vi "test pass channel to async vis.vi"(11 "Test Case In":refnum<class "Tests Event MessengerM.lvclass">) -> (0 "error out":errorcluster, 3 "Test Case Out":refnum<class "Tests Event MessengerM.lvclass">)   [LabVIEW 2020, in "Tests Event MessengerM.lvclass"]
uses:
  Tests Event MessengerM.lvclass
  C:/Program Files/National Instruments/LabVIEW 2025/vi.lib/Astemes/LUnit/Test Case.lvclass
  <vilib>/Astemes/LUnit/Test Case.lvclass/Test Case.ctl
  Tests Event MessengerM.lvclass/Tests Event MessengerM.ctl
  source/Event MessengerM.lvlib
  <vilib>/Astemes/LUnit/Test Case.lvclass
  C:/Program Files/National Instruments/LabVIEW 2025/vi.lib/Astemes/LUnit/LUnit Runnable.lvclass
  D:/git/Event-MessengerM-Channel-Wire/tests/Tests Event MessengerM/Tests Event MessengerM.lvclass
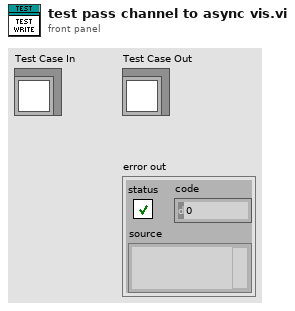
[diagram p1: front panel]
types:
  T1 = typedef "Event MessengerM.lvlib/))Channel.ctl" = refnum<queue>
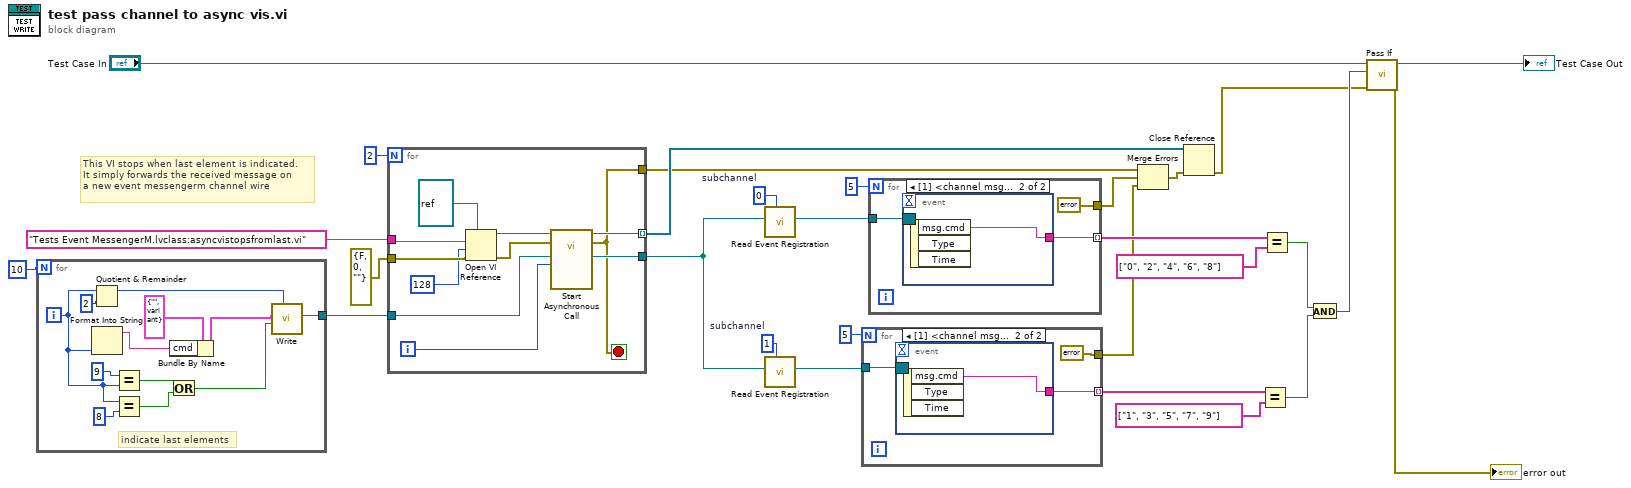
[diagram p0: block diagram]
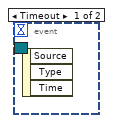
[diagram p2: hidden frame]
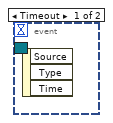
[diagram p3: hidden frame]
diagram:
  w3 = 1  # subchannel
  w4 = 0  # subchannel
  # "This VI stops when last element is indicated.\nIt simply forwards the received message on\na new event messengerm channel wire"
  n1 = for {
    N: 10 -> [_]
    tunnel: [w40] -> w12
    i -> [w30]
    # "indicate last elements"
    n2 = Quotient & Remainder(x=w30, y=2) -> (x-y*floor(x/y)=w38:i32)  [unwired: 1 out]
    n3 = Format Into String(w30) -> (resulting string=w35:string)  [unwired: 3 in, 1 out]
    n4 = Equal?(x=9, y=w30) -> (x = y?=w33:bool)
    n5 = Equal?(x=w30, y=8 ("x")) -> (x = y?=w29:bool)
    n6 = Or(x=w33, y=w29) -> (x .or. y?=w32:bool)
    n7 = Bundle By Name(cluster=cluster{"cmd":string, "data":variant} {"cmd"="", "data"=variant} ("element"), "cmd"=w35) -> (w36:cluster{"cmd":string, "data":variant})
    n8 = call "Write.vi"("subchannel (0)"=w38, "last element? (F)"=w32, "element"=w36) -> ("channel"=w40:T1)  [unwired: 7 in, 1 out]
  }
  n9 = for {
    N: 2 -> [_]
    tunnel: "Tests Event MessengerM.lvclass:asyncvistopsfromlast.vi" -> [w51]
    tunnel: w12 -> [w48]
    tunnel: errorcluster {"status"=FALSE, "code"=0, "source"=""} ("error constant") -> [w46]
    tunnel: [w45] -> w10
    tunnel: [w44] -> w5 mode=indexing
    tunnel: [w41] -> w1
    i -> [w43]
    stop <- w41 stop-if-true
    n10 = Open VI Reference(type specifier VI Refnum (for type only)=refnum<vi> refnum, vi path=w51, options=128, error in (no error)=w46) -> (vi reference=w49:refnum<vi>, error out=w47:errorcluster)  [unwired: 2 in]
    n11 = call-by-ref "Start Asynchronous Call"(reference=w49, error in=w47, "subchannel"=w43, "channel"=w48) -> (reference out=w44:refnum<vi>, error out=w41:errorcluster, "other channel out"=w45:T1)  [unwired: 9 in]
  }
  n12 = call "Read Event Registration.vi"("subchannel"=w4, "channel"=w10) -> ("event registration refnum"=w24:refnum<event-registration>)  [unwired: 9 in]
  n13 = call "Read Event Registration.vi"("subchannel"=w3, "channel"=w10) -> ("event registration refnum"=w23:refnum<event-registration>)  [unwired: 9 in]
  n14 = for {
    N: 5 -> [_]
    tunnel: w23 -> [w54]
    tunnel: [w53] -> w20 mode=indexing
    tunnel: [errorcluster {"status"=FALSE, "code"=0, "source"=""} ("error constant")] -> w8
    n15 = event shown="[1] <channel msg>: User Event" {
      selector: w54 -> [_ _]
      dyn-events: _ -> [_ _]
      timeout: _ -> [_ _]
      tunnel: [_ w55] -> w53
      event Timeout {
        n16 = event-data() -> ()  [unwired: 1 in, 3 out]
      }
      event User Event {
        n17 = event-data() -> ("msg.cmd"=w55:string)  [unwired: 1 in, 2 out]
      }
    }
  }
  n18 = for {
    N: 5 -> [_]
    tunnel: w24 -> [w58]
    tunnel: [w57] -> w17 mode=indexing
    tunnel: [errorcluster {"status"=FALSE, "code"=0, "source"=""} ("error constant")] -> w7
    n19 = event shown="[1] <channel msg>: User Event" {
      selector: w58 -> [_ _]
      dyn-events: _ -> [_ _]
      timeout: _ -> [_ _]
      tunnel: [_ w59] -> w57
      event Timeout {
        n20 = event-data() -> ()  [unwired: 1 in, 3 out]
      }
      event User Event {
        n21 = event-data() -> ("msg.cmd"=w59:string)  [unwired: 1 in, 2 out]
      }
    }
  }
  n22 = Merge Errors(w1, w7, w8) -> (w6:errorcluster)
  n23 = Close Reference(reference=w5, error in (no error)=w6) -> (error out=w2:errorcluster)
  n24 = Equal?(x=w20, y=string[] ["1", "3", "5", "7", "9"] ("Array 2")) -> (x = y?=w18:bool)
  n25 = Equal?(x=w17, y=string[] ["0", "2", "4", "6", "8"] ("Array")) -> (x = y?=w15:bool)
  n26 = And(x=w15, y=w18) -> (x .and. y?=w14:bool)
  n27 = call <vilib>:"Pass If.vi"("error in (no error)"=w2, "Pass?"=w14, "LUnit Test Case In"="Test Case In") -> ("error out"=→"error out":errorcluster, "LUnit Test Case Out"=→"Test Case Out":refnum<class "Tests Event MessengerM.lvclass">)  [unwired: 7 in]
